vi "IpDFT-only-DC_2x9215.vi"() -> ()   [LabVIEW 2021]
doc: "This example is an implementation of the FPGA part of the Phasor Measurement Unit. It performs data acquisition, timestamping based on GPS, digital filtering, decimation frequency measurement and insertion of data into DMA FIFO."
uses:
  <vilib>/eio/EIONode/EIONode.xnode
  <vilib>/Platform/TimedLoop/XDataNode/wakeup.ctl
  <vilib>/Platform/TimedLoop/XDataNode/XDNodeRunTimeDep.lvlib
  <vilib>/Platform/TimedLoop/XDataNode/nitl_modes.ctl
  <vilib>/Platform/TimedLoop/XDataNode/timing_clust.ctl
  <vilib>/Platform/TimedLoop/XDataNode/XDataNode.xnode
  <vilib>/rvi/FXPMathLib/basic elements/FxpIntAccumulator/subVIs/nifxpmath_IntAccumulator_SimConfig.ctl
  <vilib>/rvi/FXPMathLib/basic elements/FxpIntAccumulator/simVIs/DllFxpIntAccumulator_sub.vi
  <vilib>/rvi/FXPMathLib/basic elements/FxpIntAccumulator/XNode/nifxpmath_IntAccumulator.xnode
  <vilib>/rvi/FXPMathLib/FxpMul/XNode/nifxpmath_Multiplier.xnode
  <vilib>/rvi/FXPMathLib/sim/FxpSim.dll
  <vilib>/rvi/Analysis/common/codeGenErrors/XNode/niFpgaXNodeCodeGenErrorHandle.vi
  <vilib>/rvi/Analysis/measure/dc-rms/XNode/niFpgaDC-RMS.xnode
  <vilib>/rvi/FXPMathLib/FxpSqrt/XNode/nifxpmath_Sqrt.xnode
  <vilib>/rvi/FXPMathLib/FxpSqrt/simVIs/DllSqrtTemp_sub.vi
  <vilib>/fxp/LVFixedPointOverflowPolicyTypeDef.ctl
  <vilib>/rvi/FXPMathLib/FxpSqrt/subVIs/nifxpmath_Sqrt_SimConfig.ctl
  <vilib>/rvi/eio/common/nirviEmuTemplateMethod_errors.vi
panel:
  out "I_BAT1":fxp<+,20,5>
  out "V_BAT2":fxp<+,20,5>
  out "I_BAT2":fxp<+/-,20,5>
  out "V_BAT1":fxp<+/-,20,5>
  out "V_PV1":fxp<+,20,5>
  out "I_PV1":fxp<+,20,5>
  out "I_PV2":fxp<+/-,20,5>
  out "V_PV2":fxp<+/-,20,5>
  out "No. of channel":i32
  out "start index":u16[](array[numeric])
  out "Pipeline size":i32=4
  out "Pipeline ID":i32
  out "CB Size":u16
  out "N":i32
  out "iMAX":u16
  out "dF [Hz]":fxp<+,36,5>
  # "FPGA PMU EPFL/DESL"
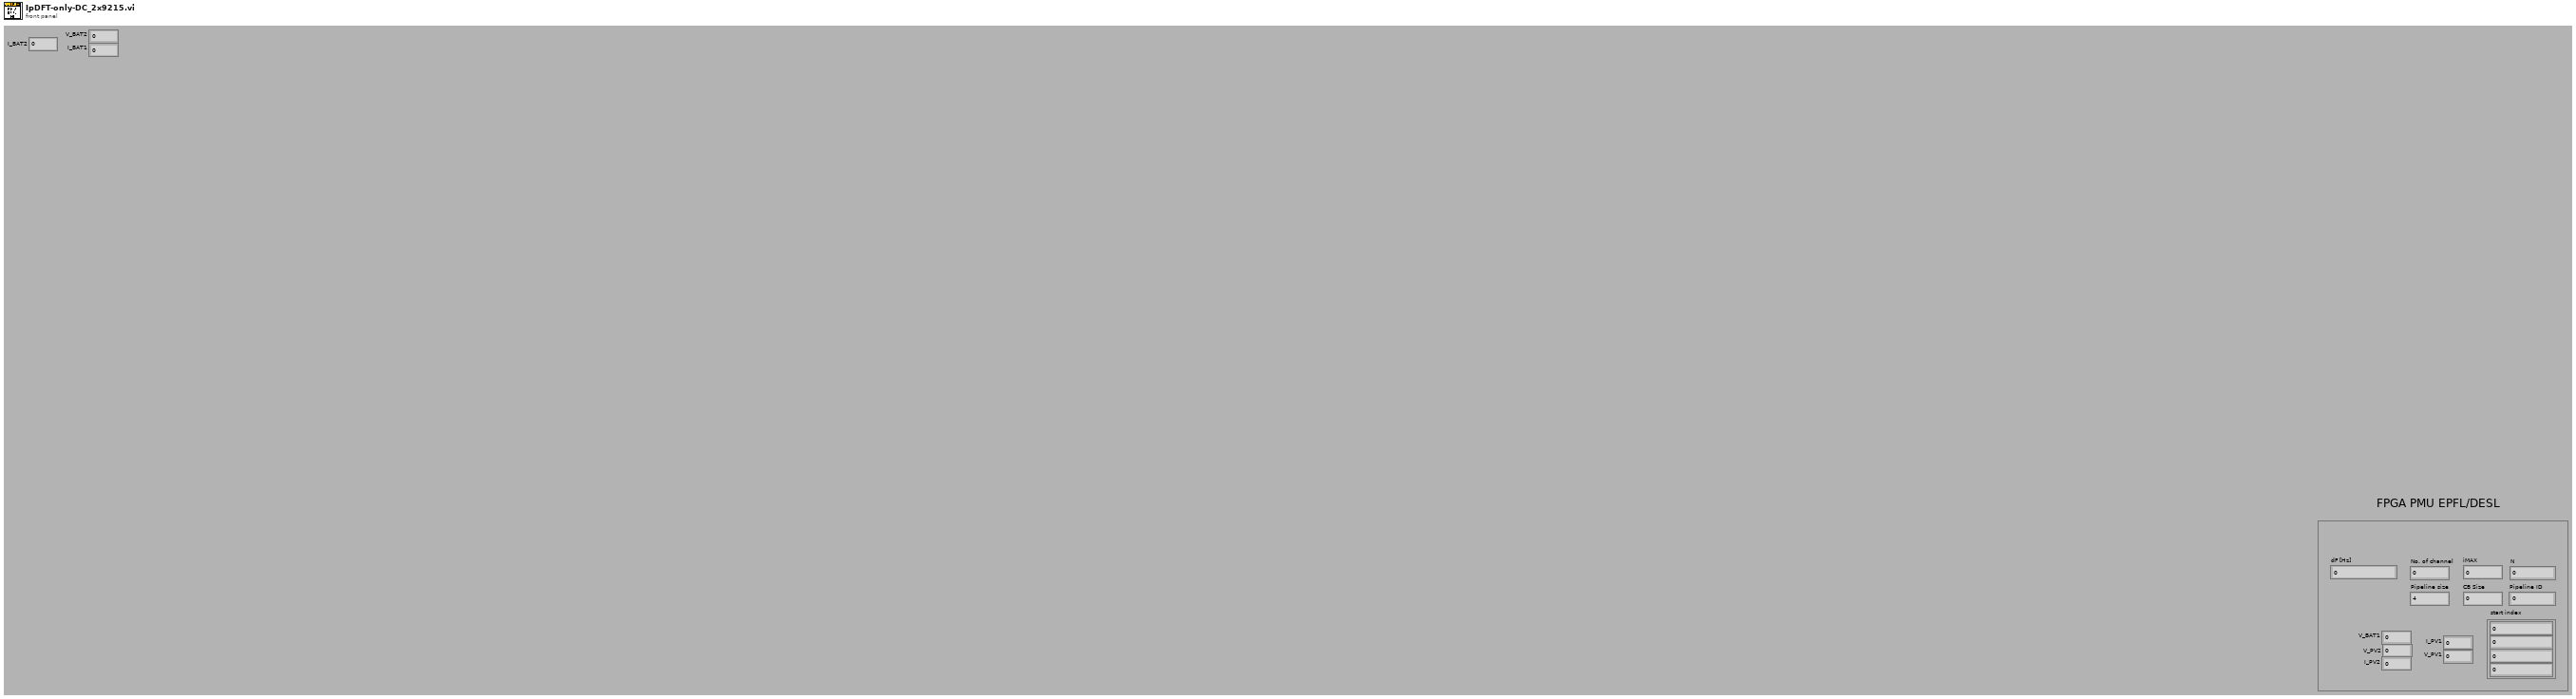
[diagram p1: front panel]
types:
  T1 = typedef "XDNodeRunTimeDep.lvlib/timing_clust.ctl" = cluster{"Expected End [f-1]":u64, "Actual End [f-1]":u64, "Finished Late? [f-1]":bool, "Expected End [i-1]":u64, "Actual End [i-1]":u64, "Finished Late? [i-1]":bool, "Expected Start [i]":u64, "Actual Start [i]":u64, "Expected Start [f]":u64, "Actual Start [f]":u64, "Source Name":string, "Structure Name":string, "Period":i64, "Deadline":i64, "Offset":i64, "Start":i64, "Priority":i32, "Timeout":i32, "Mode":T2, "Wakeup Reason":T3, "Error":errorcluster, "Source Type":string, "Secondary Source Type":string, "Global End Time":u64, "Global Start Time":u64, "Frame Duration":u64, "Iteration Duration":u64, "Assigned CPU":i32, "I/O Scan Engine Mode":u32}
  T2 = typedef "XDNodeRunTimeDep.lvlib/nitl_modes.ctl" = enum32{"No Change", "Process missed periods, maintain original phase", "Discard missed periods, maintain original phase", "Process missed periods, ignore original phase", "Discard missed periods, ignore original phase"}
  T3 = typedef "XDNodeRunTimeDep.lvlib/wakeup.ctl" = enum32{"Normal", "Aborted", "Asynchronous wakeup", "Timing source error", "Timed loop error", "Timeout"}
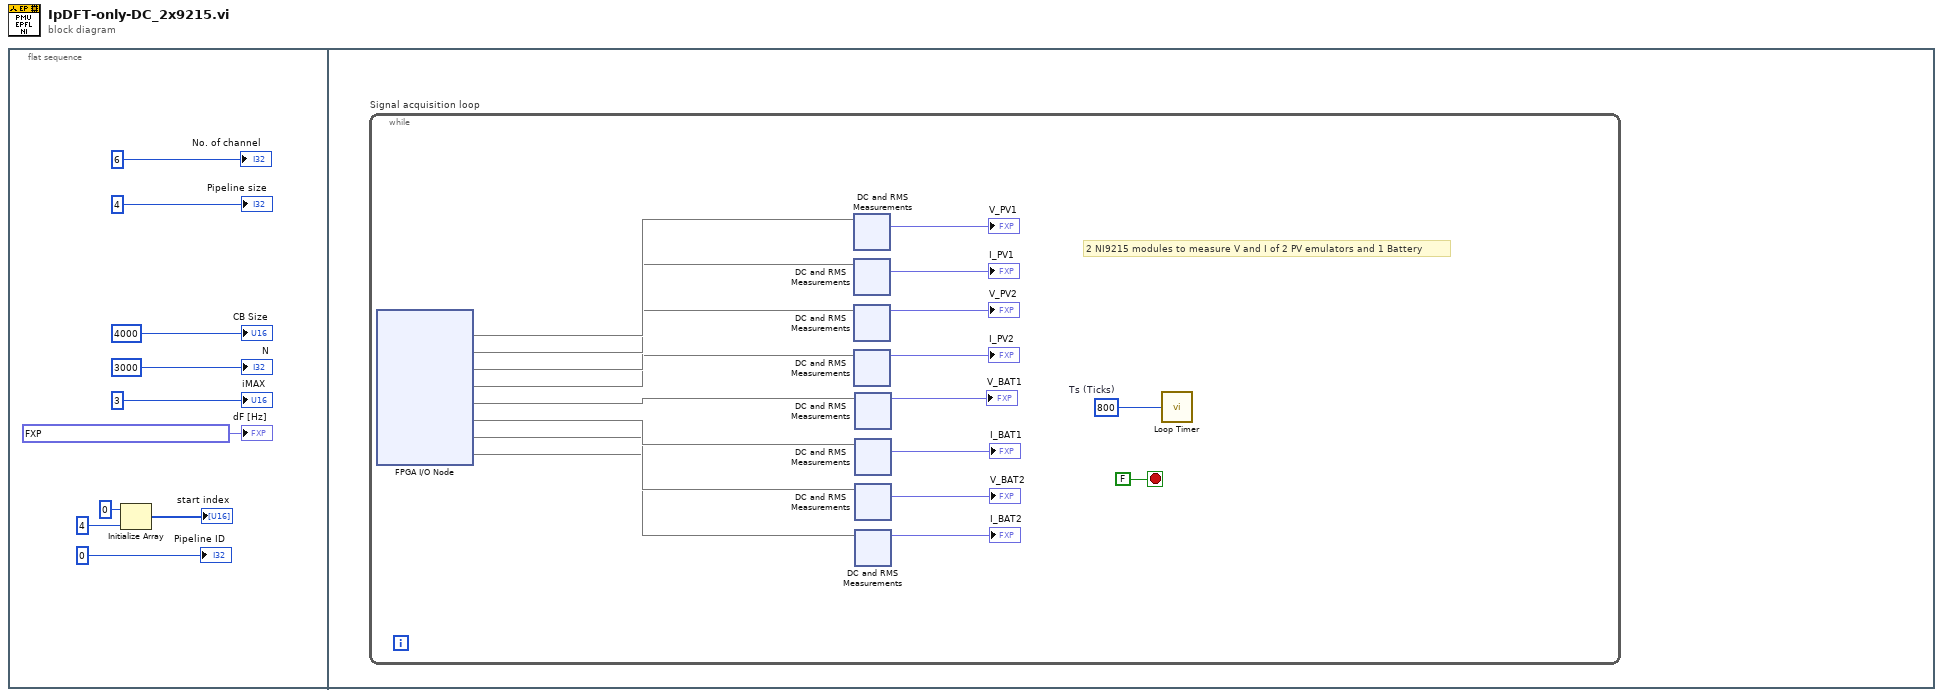
[diagram p0: block diagram]
diagram:
  n1 = flat-sequence {
    frame #0 {
      n2 = Initialize Array(u16 0 ("element"), 4 ("dimension size")) -> (→"start index":u16[])
      "dF [Hz]" <- fxp<+,36,5> 16.666666666511446 ("dF [Hz]")
      "iMAX" <- u16 3 ("samples counter 2")
      "N" <- 3000 ("Samples/ch")
      "CB Size" <- u16 4000 ("CB Size")
      "Pipeline size" <- 4 ("Pipeline size")
      "No. of channel" <- 6 ("Number of channel")
      "Pipeline ID" <- 0 ("Pipeline ID")
    }
    frame #1 {
      n3 = while "Signal acquisition loop" {
        stop <- FALSE stop-if-true
        w27 = u32 800  # Ts (Ticks)
        # "2 NI9215 modules to measure V and I of 2 PV emulators and 1 Battery"
        n4 = xnode "FPGA I/O Node"() -> ("Mod2/AI0"=w18, "Mod2/AI1"=w17, "Mod2/AI2"=w16, "Mod2/AI3"=w15, "Mod3/AI0"=w14, "Mod3/AI1"=w13, "Mod3/AI2"=w12, "Mod3/AI3"=w11)  [unwired: 8 in, 8 out]
        n5 = xnode "DC and RMS Measurements"("input data"=w18) -> ("RMS"=→"V_PV1":fxp<+,20,5>)  [unwired: 1 in, 1 out]
        n6 = xnode "DC and RMS Measurements"("input data"=w17) -> ("RMS"=→"I_PV1":fxp<+,20,5>)  [unwired: 1 in, 1 out]
        n7 = xnode "DC and RMS Measurements"("input data"=w16) -> ("DC"=→"V_PV2":fxp<+/-,20,5>)  [unwired: 1 in, 1 out]
        n8 = xnode "DC and RMS Measurements"("input data"=w15) -> ("DC"=→"I_PV2":fxp<+/-,20,5>)  [unwired: 1 in, 1 out]
        n9 = xnode "DC and RMS Measurements"("input data"=w14) -> ("DC"=→"V_BAT1":fxp<+/-,20,5>)  [unwired: 1 in, 1 out]
        n10 = xnode "DC and RMS Measurements"("input data"=w13) -> ("RMS"=→"I_BAT1":fxp<+,20,5>)  [unwired: 1 in, 1 out]
        n11 = xnode "DC and RMS Measurements"("input data"=w12) -> ("RMS"=→"V_BAT2":fxp<+,20,5>)  [unwired: 1 in, 1 out]
        n12 = xnode "DC and RMS Measurements"("input data"=w11) -> ("DC"=→"I_BAT2":fxp<+/-,20,5>)  [unwired: 1 in, 1 out]
        n13 = call "Loop Timer"("Count(Ticks)"=w27) -> ()  [unwired: 1 out]
      }
    }
  }
